vi "dvp Vi Get Gamma State.vi"(10 "pGammaState":i32, 11 "handle":u32) -> (2 "pGammaState out":i32, 3 "function return":u32(ring))   [LabVIEW 2018, in "LabViewDVPCamera.lvlib"]
doc: "LabviewDvp2Api dvpStatus dvpViGetGammaState(dvpHandle handle, BOOL *pGammaState);"
uses:
  LabViewDVPCamera.lvlib
  LabViewDVPCamera/LabViewDVPCamera.dll
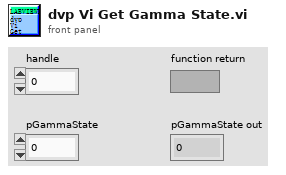
[diagram p1: front panel]
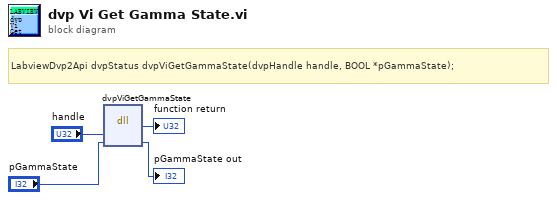
[diagram p0: block diagram]
diagram:
  # "LabviewDvp2Api dvpStatus dvpViGetGammaState(dvpHandle handle, BOOL *pGammaState);"
  n1 = dll-call lib="C:/Program Files (x86)/DVP2 Labview cn 64/Sample/LabViewDVPCamera/LabViewDVPCamera.*" fn="dvpViGetGammaState"("handle"="handle", "pGammaState"="pGammaState") -> (→"function return":u32, "pGammaState"=→"pGammaState out":i32)  [unwired: 4 in, 2 out]
